vi "Get Waypoint.vi"(8 "error in":errorcluster, 10 "System":string, 11 "Data Cluster in":T1) -> (0 "error out":errorcluster, 2 "Response body":string, 3 "Data Cluster out":T1)   [LabVIEW 2024, in "GUI.lvlib" / "Functions.lvlib"]
uses:
  Functions.lvlib
  Module Data--cluster.ctl
  <vilib>/addons/_JKI.lib/REST Client/classes/REST Client/REST Client.lvclass
  GUI.lvlib
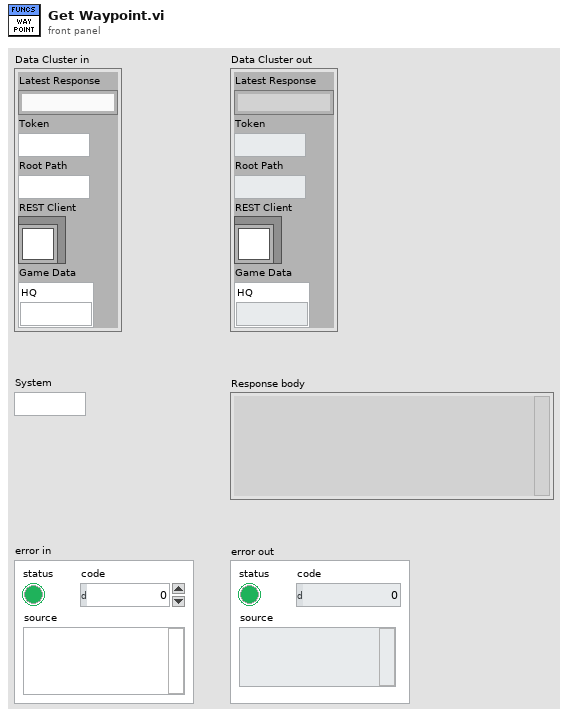
[diagram p1: front panel]
types:
  T1 = typedef "GUI.lvlib/Module Data--cluster.ctl" = cluster{"Latest Response":string, "Token":string, "Root Path":string, "REST Client":refnum<class "REST Client.lvclass">, "Game Data":cluster{"HQ":string}}
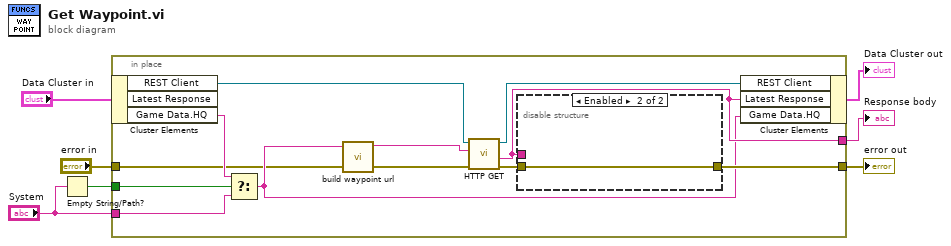
[diagram p0: block diagram]
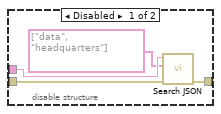
[diagram p2: hidden frame]
diagram:
  n1 = Empty String/Path?(string/path="System") -> (empty?=w3:bool)
  n2 = in-place {
    in-place-border: [w15] -> w4
    in-place-border: [w16] -> w5
    in-place-border: w3 -> [w12]
    in-place-border: "System" -> [w10]
    in-place-border: "error in" -> [w8]
    n3 = in-place-cluster #1("Data Cluster in") -> ("REST Client"=w19:refnum<class "REST Client.lvclass">, "Game Data.HQ"=w11:string)  [unwired: 1 out]
    n4 = Select(t=w11, s=w12, f=w10) -> (s? t:f=w9:string)
    n5 = call "build waypoint url.vi"("error in (no error)"=w8, "System"=w9) -> ("error out"=w13:errorcluster, "url"=w14:string)  [unwired: 8 in]
    n6 = call-dynamic "HTTP GET.vi"("error in (no error)"=w13, "Path"=w14, "REST Client in"=w19) -> ("error out"=w17:errorcluster, "Response body"=w16:string, "REST Client out"=w18:refnum<class "REST Client.lvclass">)  [unwired: 3 in, 3 out]
    n7 = disable-structure shown="Enabled" {
      disable-tunnel: w17 -> [w23 w24]
      disable-tunnel: w16 -> [w22 _]
      disable-tunnel: [w21 w24] -> w15
      frame Disabled {
        n8 = call "Search JSON.vi"("error in"=w23, "Name Array 2"=string[] ["data", "headquarters"] ("Name Array"), "Response body"=w22) -> ("error out"=w21:errorcluster)  [unwired: 7 in, 1 out]
      }
      frame Enabled {
      }
    }
    n9 = in-place-cluster #1("REST Client"=w18, "Latest Response"=w16, "Game Data.HQ"=w9) -> (→"Data Cluster out":T1)
  }
  "error out" <- w4
  "Response body" <- w5
